vi "magTerm_TREEstate.vi"() -> ()   [LabVIEW 2014]
uses:
  <vilib>/Utility/file.llb/Read From Spreadsheet File (string).vi
  common/crest/LabVIEW/LV14/libcommon-crest.lvlib
panel:
  out "Waveform Chart":dbl[][](graph)
  out "current_buffer_array":dbl[][](array[numeric])
  out "array (last n elements first)":dbl[](array[numeric])
  in  "Tab Control":enum32{"Page 1", "Page 2"}(tab)
  out "handle":u32
  in  "Simulated/real":string(combo)="BTF_SIM"
  in  "Set_prog_state":bool
  in  "file path (dialog if empty)":path
  out "file_data":string[][](array[string])
  in  "stop":bool
  in  "!CHAOS WAN url":string="192.168.150.91:8081"
  out "Set_prog_Current":string[](array[string])
  out "RUN":bool
  out "Element List":string[](array[string])
  in  "buffer_size":i32=100
  out "function return":i32
  out "error":u32
  out "set_current_new":dbl
  out "set_current_new_control":string
  out "Array Element.Value":variant
  out "Timeout_Array":i64[](array[numeric])
  in  "Single MAG SETUP":T1
  out "MAG array display":T2(array[cluster])
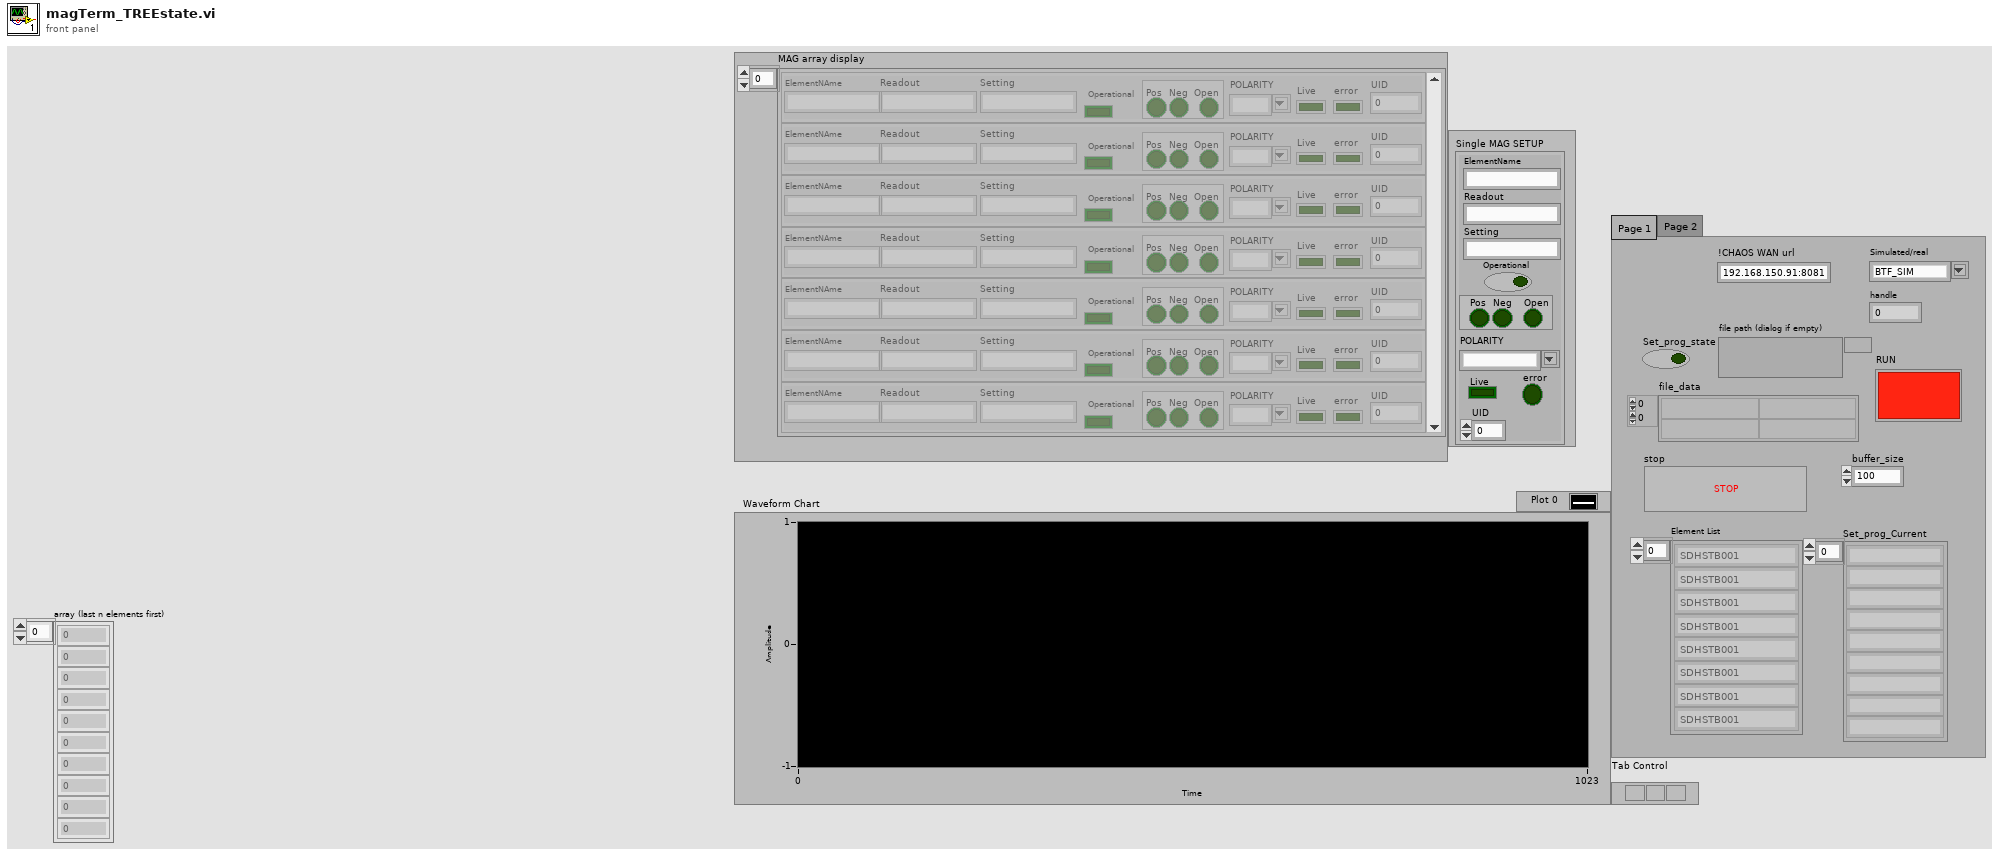
[diagram p1: front panel]
types:
  T1 = cluster{"ElementName":string, "Readout":string, "Setting":string, "Operational":bool, "Pos":bool, "Neg ":bool, "Open":bool, "Live":bool, "error":bool, "UID":u32, "POLARITY":string}
  T2 = cluster{"ElementNAme":string, "Readout":string, "Setting":string, "Operational":bool, "Pos":bool, "Neg ":bool, "Open":bool, "Live":bool, "error":bool, "UID":u32, "POLARITY":string}[]
  T3 = cluster{"ElementName":string, "Readout":string, "Setting":string, "Operational":bool, "Pos":bool, "Neg ":bool, "Open":bool, "Live":bool, "error":bool, "UID":u32, "POLARITY":string}[]
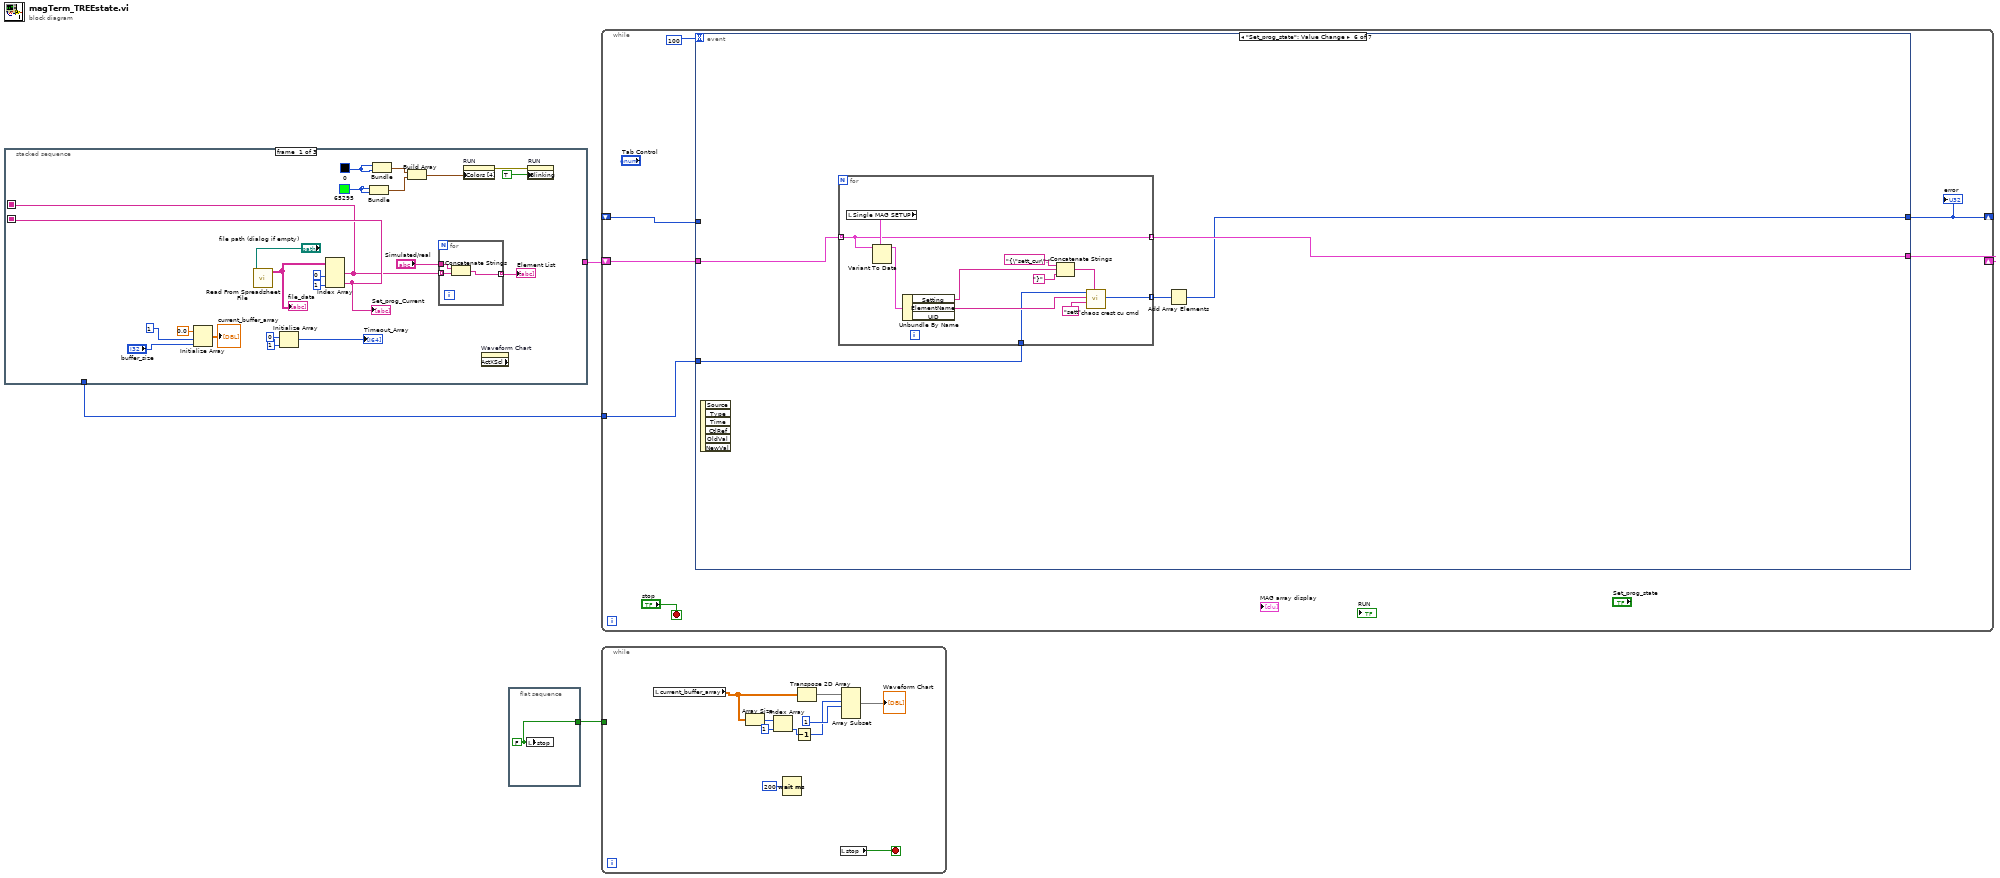
[diagram p0: block diagram]
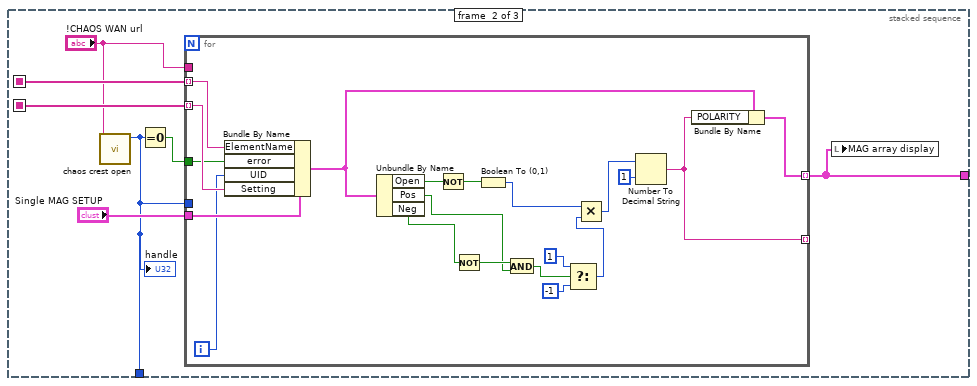
[diagram p2: hidden frame]
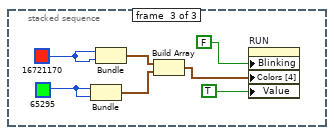
[diagram p3: hidden frame]
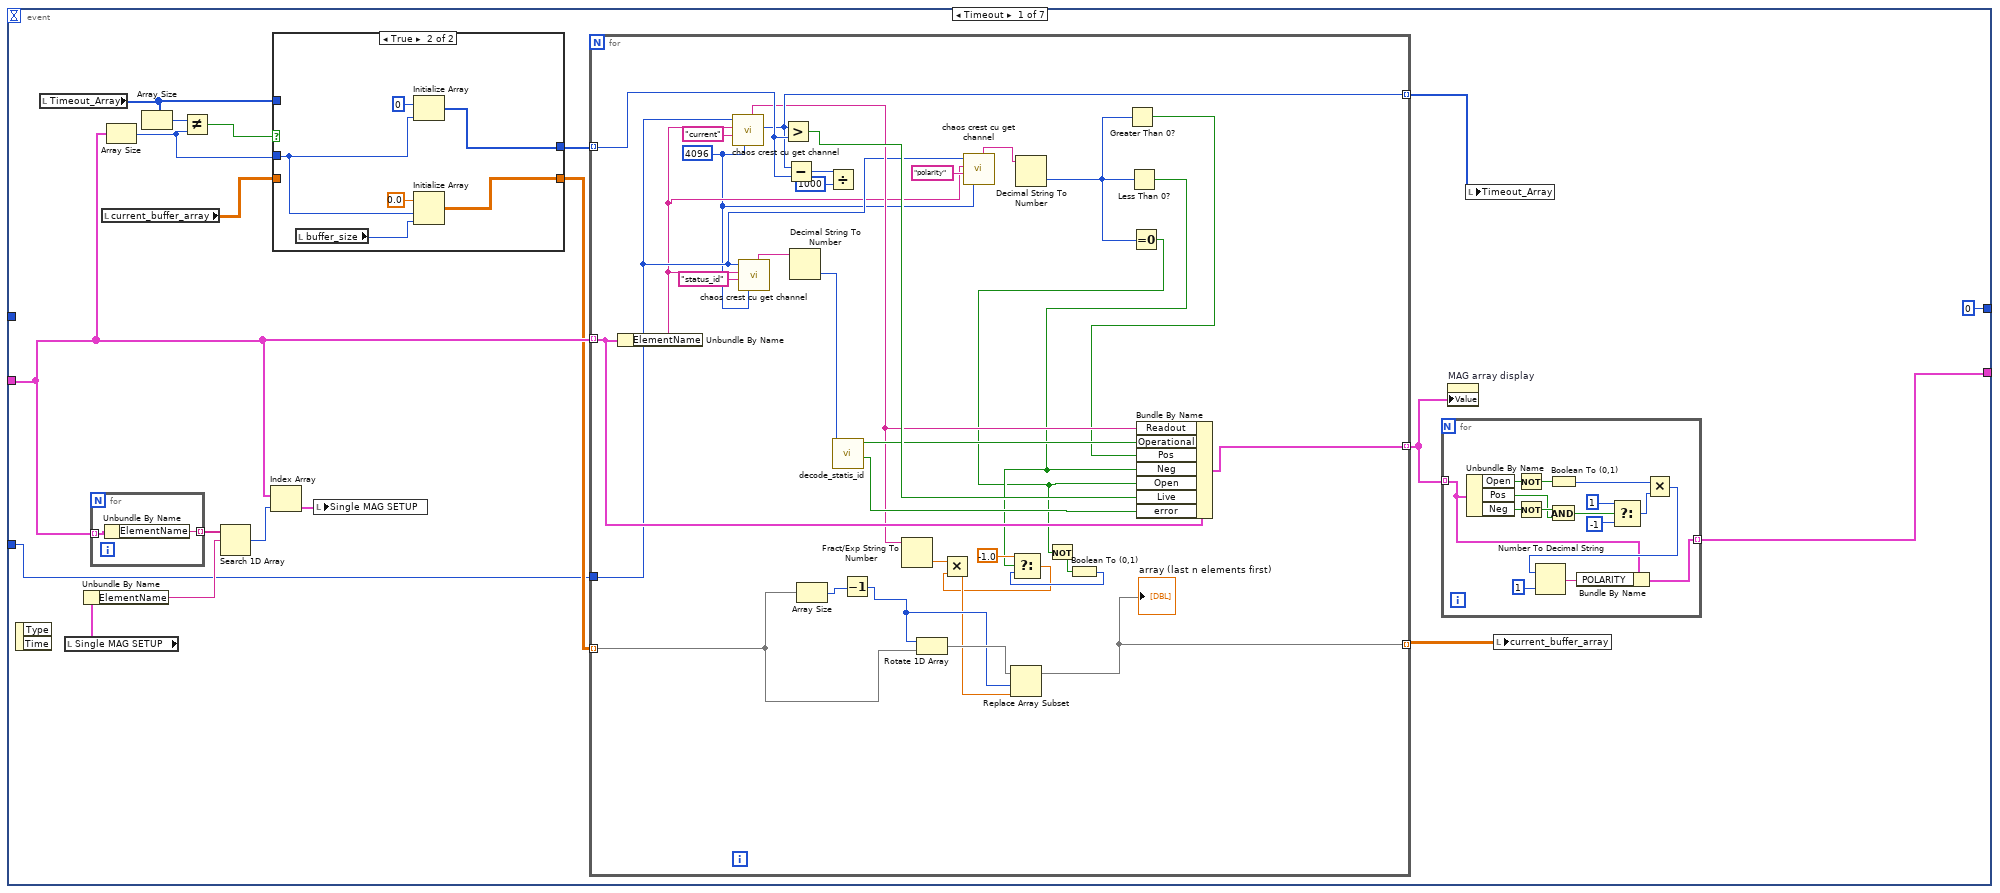
[diagram p4: hidden frame]
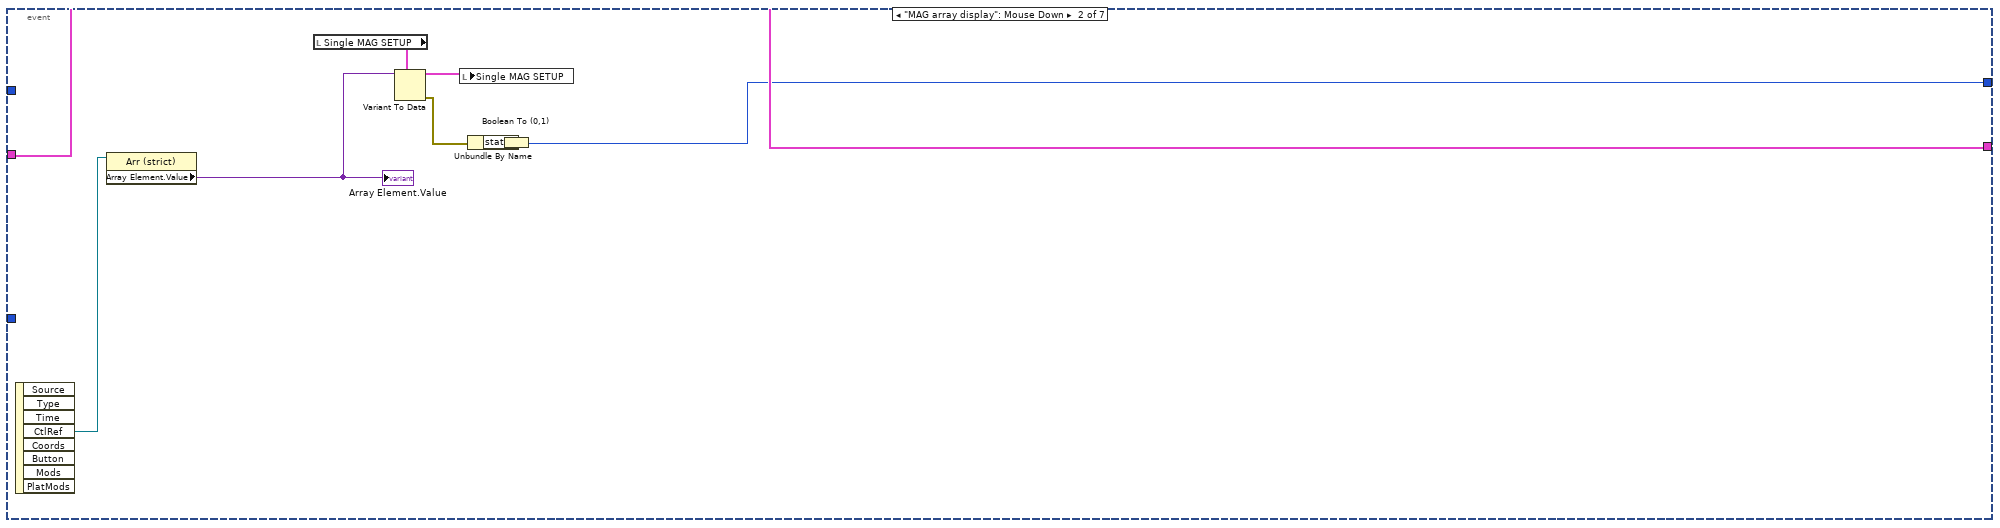
[diagram p6: hidden frame]
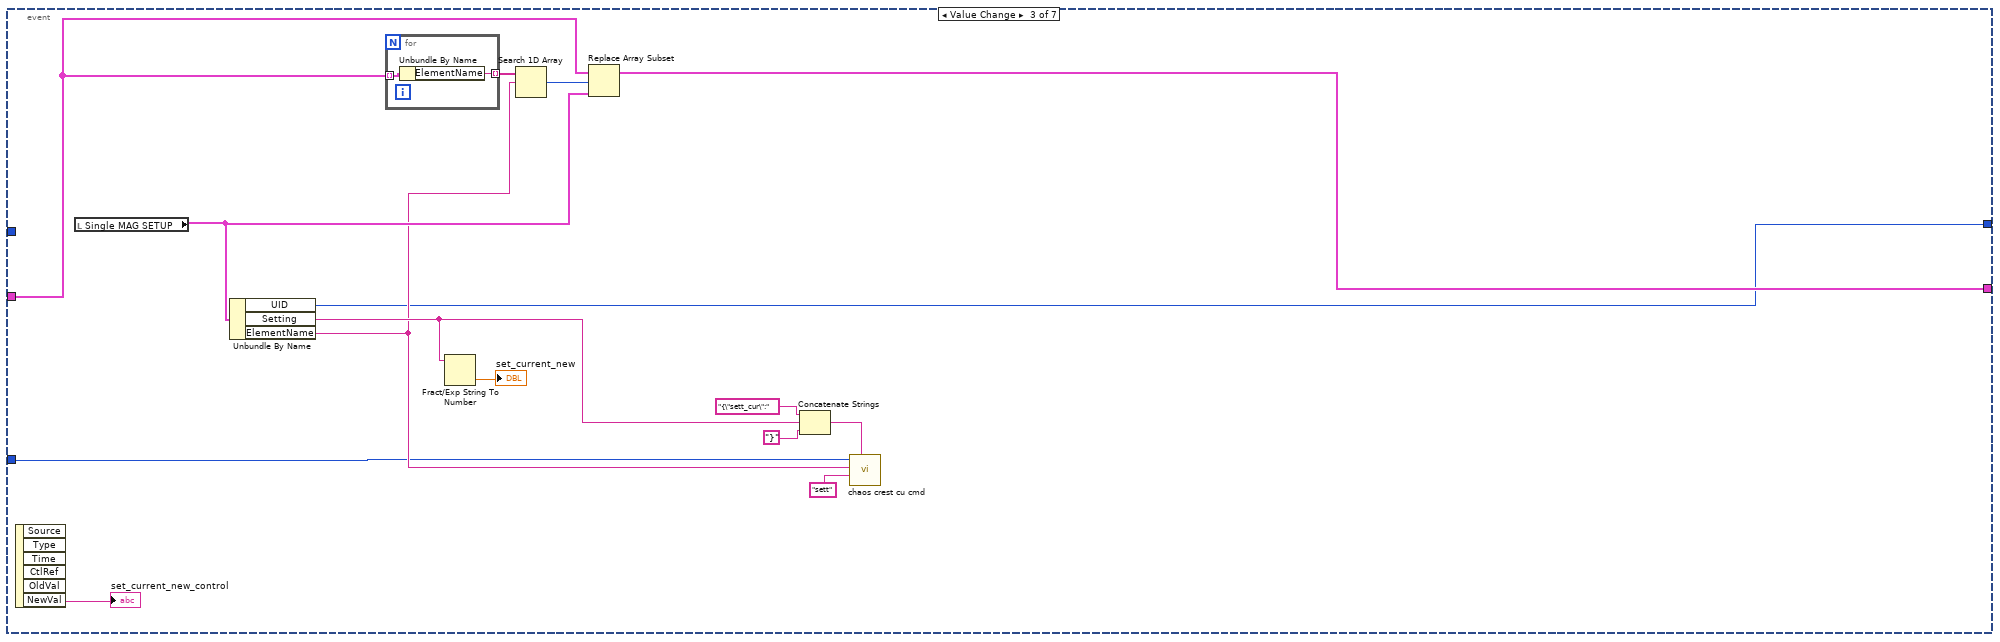
[diagram p7: hidden frame]
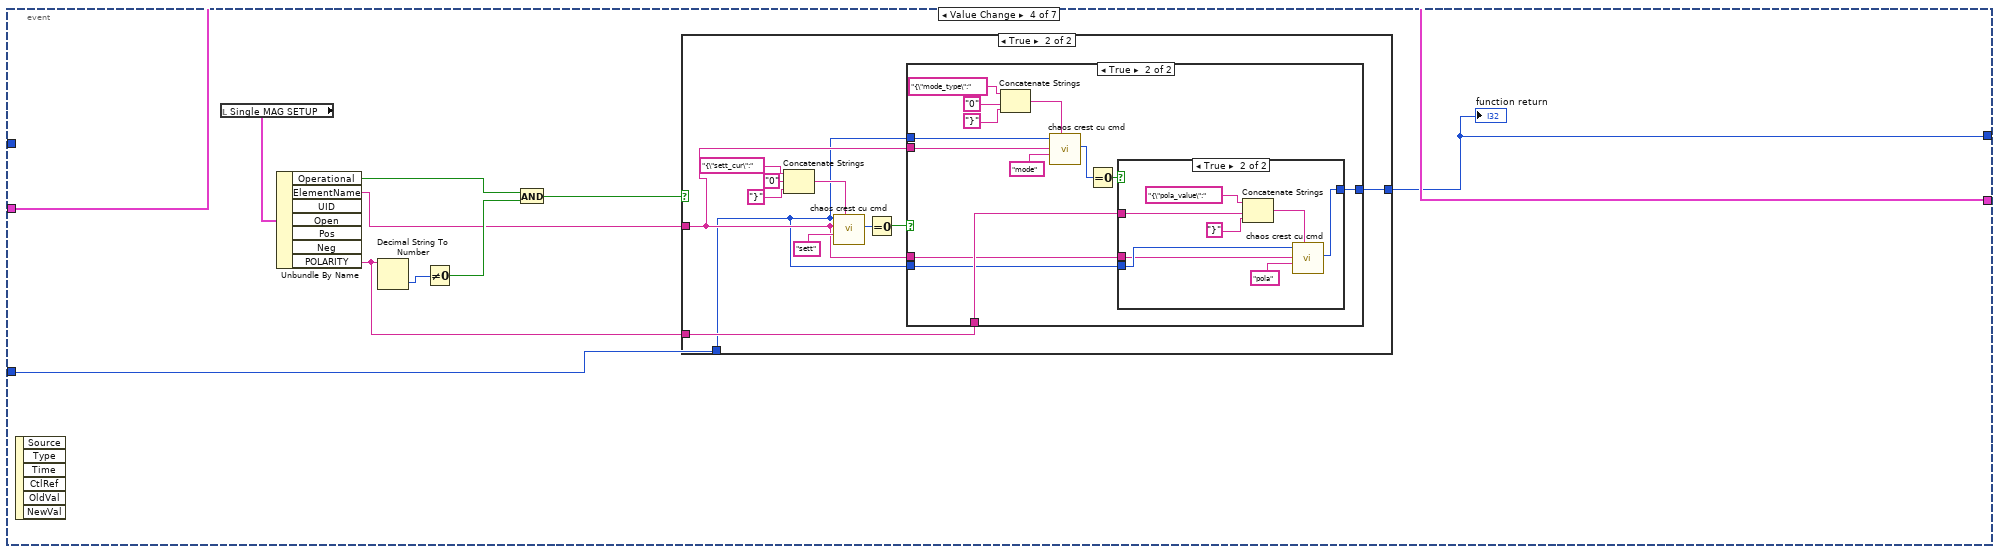
[diagram p8: hidden frame]
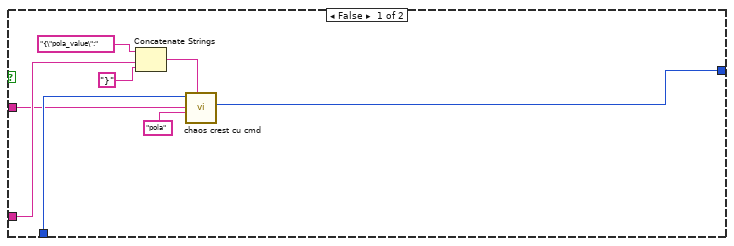
[diagram p9: hidden frame]
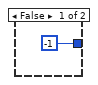
[diagram p10: hidden frame]
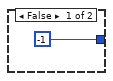
[diagram p11: hidden frame]
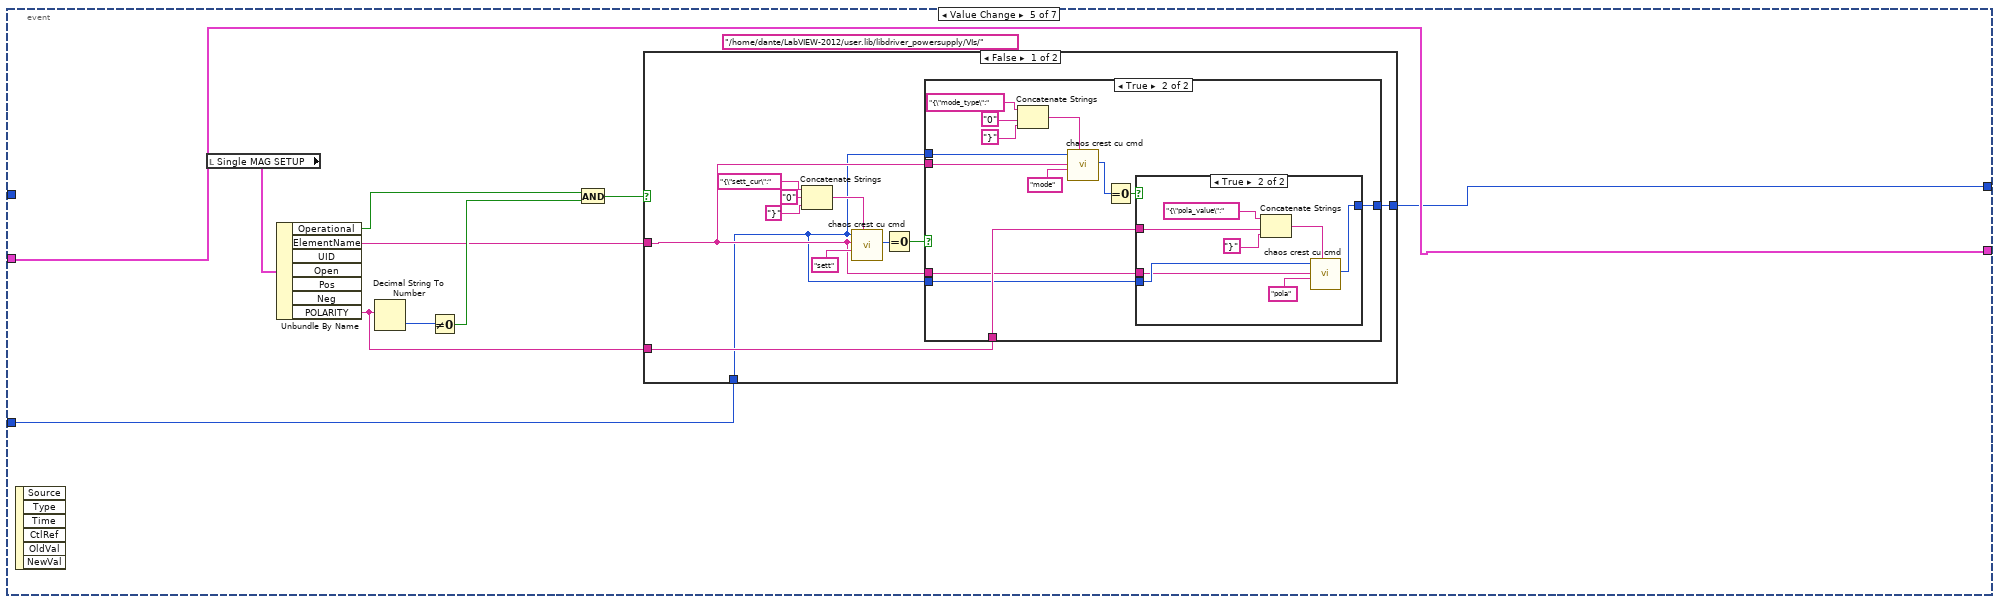
[diagram p12: hidden frame]
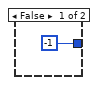
[diagram p13: hidden frame]
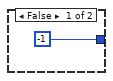
[diagram p14: hidden frame]
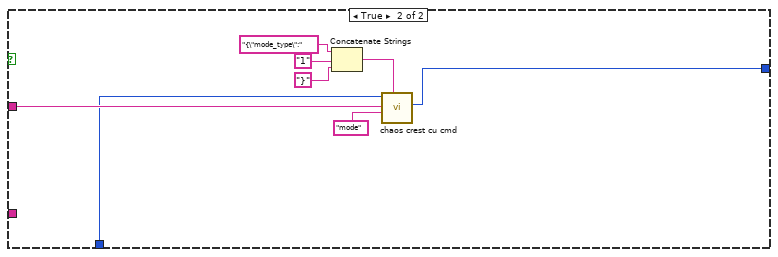
[diagram p15: hidden frame]
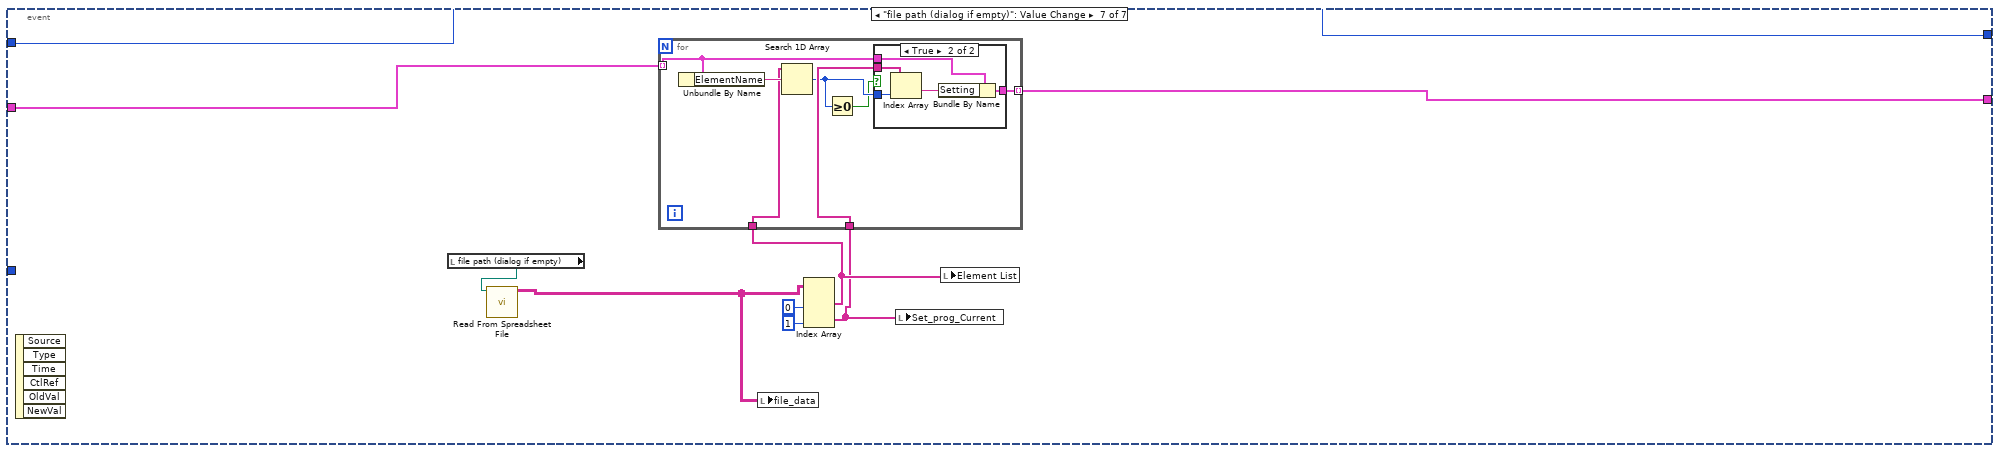
[diagram p16: hidden frame]
diagram:
  n1 = stacked-sequence {
    seq-local: [w6 _ _] -> [_ w35 _]
    seq-local: [w21 _ _] -> [_ w34 _]
    tunnel: [_ w33 _] -> w3
    tunnel: [_ w29 _] -> w1
    frame #0 {
      w17 = u32 0
      w16 = u32 65295
      n2 = Initialize Array(0.0 ("element"), 1 ("dimension size"), "buffer_size") -> (→"current_buffer_array":dbl[][])
      n3 = call-poly <vilib>:"Read From Spreadsheet File.vi"("file path (dialog if empty)"="file path (dialog if empty)") -> ("all rows"=w24:string[][])  [unwired: 6 in, 4 out]
      "file_data" <- w24
      n4 = Initialize Array(i64 0 ("element"), 1 ("dimension size")) -> (→"Timeout_Array":i64[])
      n5 = Index Array(array=w24, index (col) #1=0 ("disabled index (col)"), index (col) #2=1 ("index (col)")) -> (element #1=w6:string[], element #2=w21:string[])  [unwired: 2 in]
      "Set_prog_Current" <- w21
      n6 = Bundle(w16, w16) -> (w19:cluster{u32, u32})  [unwired: 1 in]
      n7 = Bundle(w17, w17) -> (w20:cluster{u32, u32})  [unwired: 1 in]
      n8 = Build Array(w20, w19) -> (w18:cluster{u32, u32}[])
      n9 = for {
        tunnel: w6 -> [w28] mode=indexing
        tunnel: "Simulated/real" -> [w27]
        tunnel: [w26] -> w4 mode=indexing
        n10 = Concatenate Strings(w27, w28) -> (w26:string)
      }
      "Element List" <- w4
      n11 = property on="RUN" class="Bool (strict)"("Colors [4]"=w18) -> (error out=w12:errorcluster)  [unwired: 2 in, 1 out]
      n12 = property on="Waveform Chart" class="WFChart (strict)" props=["ActXScl"]() -> ()  [unwired: 2 in, 3 out]
      n13 = property on="RUN" class="Bool (strict)"(error in=w12, "Blinking"=TRUE) -> ()  [unwired: 1 in, 2 out]
    }
    frame #1 {
      n14 = call "chaos crest open.vi"("chaoswanurl"="!CHAOS WAN url") -> ("function return"=w29:u32)  [unwired: 10 in]
      "handle" <- w29
      n15 = Equal To 0?(x=w29) -> (x = 0?=w30:bool)
      n16 = for {
        tunnel: w35 -> [w55] mode=indexing
        tunnel: "!CHAOS WAN url" -> [_]
        tunnel: [w39] -> w33 mode=indexing
        tunnel: w34 -> [w54] mode=indexing
        tunnel: "Single MAG SETUP" -> [w53]
        tunnel: [w38] -> _ mode=indexing
        tunnel: w30 -> [w36]
        tunnel: w29 -> [_]
        i -> [w37]
        n17 = Bundle By Name(cluster=w53, "ElementName"=w55, "error"=w36, "UID"=w37, "Setting"=w54) -> (w42:T1)
        n18 = Unbundle By Name(w42) -> ("Open"=w48:bool, "Pos"=w47:bool, "Neg"=w46:bool)
        n19 = Not(x=w48) -> (.not. x?=w45:bool)
        n20 = Not(x=w46) -> (.not. x?=w52:bool)
        n21 = Boolean To (0,1)(Boolean=w45) -> (0, 1=w44:i16)
        n22 = And(x=w52, y=w47) -> (x .and. y?=w51:bool)
        n23 = Select(t=1 ("pol"), s=w51, f=-1 ("pol")) -> (s? t:f=w43:i32)
        n24 = Multiply(x=w44, y=w43) -> (x*y=w41:i32)
        n25 = Number To Decimal String(number=w41, width (-)=i16 1) -> (decimal integer string=w38:string)
        n26 = Bundle By Name(cluster=w42, "POLARITY"=w38) -> (w39:T1)
      }
      n27 = local write "MAG array display"(w33) -> ()
    }
    frame #2 {
      w56 = u32 16721170
      w57 = u32 65295
      n28 = Bundle(w57, w57) -> (w61:cluster{u32, u32})  [unwired: 1 in]
      n29 = Bundle(w56, w56) -> (w62:cluster{u32, u32})  [unwired: 1 in]
      n30 = Build Array(w62, w61) -> (w60:cluster{u32, u32}[])
      n31 = property on="RUN" class="Bool (strict)"("Blinking"=FALSE, "Colors [4]"=w60, "Value"=TRUE) -> ()  [unwired: 2 in, 2 out]
    }
  }
  n32 = flat-sequence {
    tunnel: [w63] -> w2
    frame #0 {
      w63 = FALSE ("stop")
      n33 = local write "stop"(w63) -> ()
    }
  }
  n34 = while {
    shift-right: [w67] -> _
    shift-left: w3 -> [w68]
    shift-right: [w66] -> _
    shift-left: _ -> [w65]
    tunnel: w1 -> [w64]
    stop <- "stop" stop-if-true
    n35 = event shown="[5] \"Set_prog_state\": Value Change" {
      selector: _ -> [_ _ _ _ _ _ _]
      dyn-events: _ -> [_ _ _ _ _ _ _]
      timeout: 100 -> [_ _ _ _ _ _ _]
      tunnel: w68 -> [w80 w153 w168 w181 w233 w279 w299]
      tunnel: [w76 w153 w167 w181 w233 w282 w295] -> w67
      tunnel: [u32 0 ("UID") w149 w157 w180 w232 w280 w294] -> w66
      tunnel: w65 -> [_ _ _ _ _ _ w294]
      tunnel: w64 -> [w72 _ w158 w175 w227 w278 _]
      event Timeout {
        n36 = event-data() -> ()  [unwired: 1 in, 2 out]
        n37 = local read "Timeout_Array"() -> (w88:i64[])
        n38 = local read "Single MAG SETUP"() -> (w83:T1)
        n39 = Unbundle By Name(w83) -> ("ElementName"=w81:string)
        n40 = for {
          tunnel: w80 -> [w106] mode=indexing
          tunnel: [w105] -> w82 mode=indexing
          n41 = Unbundle By Name(w106) -> ("ElementName"=w105:string)
        }
        n42 = local read "current_buffer_array"() -> (w73:dbl[][])
        n43 = Array Size(array=w80) -> (size(s)=w85:i32)
        n44 = Array Size(array=w88) -> (size(s)=w87:i32)
        n45 = Not Equal?(x=w87, y=w85) -> (x != y?=w86:bool)
        n46 = Search 1D Array(1D array=w82, element=w81) -> (index of element=w79:i32)  [unwired: 1 in]
        n47 = Index Array(array=w80, index=w79) -> (element=w78:T1)
        n48 = case shown="True" w86 {
          tunnel: w88 -> [w108 _]
          tunnel: w85 -> [_ w110]
          tunnel: [w108 w113] -> w84
          tunnel: [w107 w111] -> w75
          tunnel: w73 -> [w107 _]
          frame False {
          }
          frame True {
            n49 = local read "buffer_size"() -> (w109:i32)
            n50 = Initialize Array(i64 0 ("element"), w110) -> (w113:i64[])
            n51 = Initialize Array(0.0 ("element"), w110, w109) -> (w111:dbl[][])
          }
        }
        n52 = local write "Single MAG SETUP"(w78) -> ()
        n53 = for {
          tunnel: w80 -> [w148] mode=indexing
          tunnel: [w147] -> w77 mode=indexing
          tunnel: [w132] -> w89 mode=indexing
          tunnel: w84 -> [w133] mode=indexing
          tunnel: w75 -> [w143] mode=indexing
          tunnel: [w142] -> w74 mode=indexing
          tunnel: w72 -> [w120]
          w118 = 4096 ("maxsize")
          n54 = Unbundle By Name(w148) -> ("ElementName"=w119:string)
          n55 = call "chaos crest cu get channel.vi"("maxsize"=w118, "channame"="current", "cuname"=w119, "h"=w120) -> ("timestamp"=w132:u64, "output out"=w125:string)  [unwired: 5 in, 1 out]
          n56 = call "chaos crest cu get channel.vi"("maxsize"=w118, "channame"="status_id", "cuname"=w119, "h"=w120) -> ("output out"=w130:string)  [unwired: 5 in, 2 out]
          n57 = Greater?(x=w132, y=w133) -> (0:w131:bool)
          n58 = Subtract(x=w132, y=w133) -> (x-y=w135:u64)
          n59 = Decimal String To Number(string=w130) -> (number=w128:i32)  [unwired: 2 in, 1 out]
          n60 = Array Size(array=w143) -> (size(s)=w146:i32)
          n61 = Divide(x=w135, y=u32 1000) -> ()  [unwired: 1 out]
          n62 = call "decode_statis_id.vi"("satatus_id"=w128) -> ("Error"=w126:bool, "Operational"=w127:bool)  [unwired: 7 in, 2 out]
          n63 = Decrement(x=w146) -> (x-1=w144:i32)
          n64 = Fract/Exp String To Number(string=w125) -> (number=w124:dbl)  [unwired: 3 in, 1 out]
          n65 = Rotate 1D Array(1:w143, 2:w144) -> (0:w145:dbl[])
          n66 = call "chaos crest cu get channel.vi"("maxsize"=w118, "channame"="polarity", "cuname"=w119, "h"=w120) -> ("output out"=w122:string)  [unwired: 5 in, 2 out]
          n67 = Decimal String To Number(string=w122) -> (number=w123:i32)  [unwired: 2 in, 1 out]
          n68 = Greater Than 0?(x=w123) -> (x > 0?=w117:bool)
          n69 = Less Than 0?(x=w123) -> (x < 0?=w116:bool)
          n70 = Equal To 0?(x=w123) -> (x = 0?=w115:bool)
          n71 = Not(x=w115) -> (.not. x?=w139:bool)
          n72 = Boolean To (0,1)(Boolean=w139) -> (0, 1=w138:i16)
          n73 = Select(t=-1.0, s=w116, f=w138) -> (s? t:f=w137:dbl)
          n74 = Multiply(x=w124, y=w137) -> (x*y=w141:dbl)
          n75 = Replace Array Subset(array=w145, new element=w141, index=w144) -> (w142:dbl[])
          "array (last n elements first)" <- w142
          n76 = Bundle By Name(cluster=w148, "Readout"=w125, "Operational"=w127, "Pos"=w117, "Neg"=w116, "Open"=w115, "Live"=w131, "error"=w126) -> (w147:T1)
        }
        n77 = for {
          tunnel: [w92] -> w76 mode=indexing
          tunnel: w77 -> [w90] mode=indexing
          n78 = Unbundle By Name(w90) -> ("Open"=w100:bool, "Pos"=w99:bool, "Neg"=w98:bool)
          n79 = Not(x=w100) -> (.not. x?=w97:bool)
          n80 = Not(x=w98) -> (.not. x?=w104:bool)
          n81 = Boolean To (0,1)(Boolean=w97) -> (0, 1=w96:i16)
          n82 = And(x=w104, y=w99) -> (x .and. y?=w103:bool)
          n83 = Select(t=1 ("pol"), s=w103, f=-1 ("pol")) -> (s? t:f=w95:i32)
          n84 = Multiply(x=w96, y=w95) -> (x*y=w94:i32)
          n85 = Number To Decimal String(number=w94, width (-)=i16 1) -> (decimal integer string=w91:string)
          n86 = Bundle By Name(cluster=w90, "POLARITY"=w91) -> (w92:T1)
        }
        n87 = property on="MAG array display" class="Arr (strict)"("Value"=w77) -> ()  [unwired: 2 in, 2 out]
        n88 = local write "Timeout_Array"(w89) -> ()
        n89 = local write "current_buffer_array"(w74) -> ()
      }
      event "MAG array display": Mouse Down {
        n90 = event-data() -> ("CtlRef"=w156:refnum<vi>)  [unwired: 1 in, 7 out]
        n91 = property class="Arr (strict)"(reference=w156) -> ("Array Element.Value"=w155:variant)  [unwired: 1 in, 2 out]
        "Array Element.Value" <- w155
        n92 = local read "Single MAG SETUP"() -> (w154:T1)
        n93 = Variant To Data(type=w154, Variant=w155) -> (data=w152:T1, error out=w151:errorcluster)  [unwired: 1 in]
        n94 = local write "Single MAG SETUP"(w152) -> ()
        n95 = Unbundle By Name(w151) -> ("status"=w150:bool)
        n96 = Boolean To (0,1)(Boolean=w150) -> (0, 1=w149:i16)
      }
      event "Single MAG SETUP.Setting": Value Change {
        n97 = event-data() -> ("NewVal"=→"set_current_new_control":string)  [unwired: 1 in, 5 out]
        n98 = local read "Single MAG SETUP"() -> (w166:T1)
        n99 = Unbundle By Name(w166) -> ("UID"=w157:u32, "Setting"=w160:string, "ElementName"=w159:string)
        n100 = for {
          tunnel: w168 -> [w173] mode=indexing
          tunnel: [w172] -> w170 mode=indexing
          n101 = Unbundle By Name(w173) -> ("ElementName"=w172:string)
        }
        n102 = Fract/Exp String To Number(string=w160) -> (number=→"set_current_new":dbl)  [unwired: 3 in, 1 out]
        n103 = Search 1D Array(1D array=w170, element=w159) -> (index of element=w169:i32)  [unwired: 1 in]
        n104 = Replace Array Subset(array=w168, new element=w166, index=w169) -> (w167:T3)
        n105 = Concatenate Strings("{\"sett_cur\":", w160, "}" ("string")) -> (w163:string)
        n106 = call "chaos crest cu cmd.vi"("args"=w163, "cmd"="sett", "cuname"=w159, "h"=w158) -> ()  [unwired: 6 in, 2 out]
      }
      event "Single MAG SETUP.POLARITY": Value Change {
        n107 = event-data() -> ()  [unwired: 1 in, 6 out]
        n108 = local read "Single MAG SETUP"() -> (w183:T1)
        n109 = Unbundle By Name(w183) -> ("Operational"=w182:bool, "ElementName"=w176:string, "POLARITY"=w174:string)  [unwired: 4 out]
        n110 = Decimal String To Number(string=w174) -> (number=w179:i32)  [unwired: 2 in, 1 out]
        n111 = Not Equal To 0?(x=w179) -> (x != 0?=w178:bool)
        n112 = And(x=w182, y=w178) -> (x .and. y?=w177:bool)
        n113 = case shown="True" w177 {
          tunnel: [w184 w202] -> w180
          tunnel: w176 -> [w185 w193]
          tunnel: w175 -> [w186 w192]
          tunnel: w174 -> [w187 w194]
          frame False {
            n114 = Concatenate Strings("{\"pola_value\":", w187, "}" ("string")) -> (w190:string)
            n115 = call "chaos crest cu cmd.vi"("args"=w190, "cmd"="pola", "cuname"=w185, "h"=w186) -> ("function return"=w184:i32)  [unwired: 6 in, 1 out]
          }
          frame True {
            n116 = Concatenate Strings("{\"sett_cur\":", "0" ("string"), "}" ("string")) -> (w200:string)
            n117 = call "chaos crest cu cmd.vi"("args"=w200, "cmd"="sett", "cuname"=w193, "h"=w192) -> ("function return"=w196:i32)  [unwired: 6 in, 1 out]
            n118 = Equal To 0?(x=w196) -> (x = 0?=w195:bool)
            n119 = case shown="True" w195 {
              tunnel: [-1 ("function return") w215] -> w202
              tunnel: w194 -> [_ w214]
              tunnel: w192 -> [_ w213]
              tunnel: w193 -> [_ w212]
              tunnel: w193 -> [_ w205]
              tunnel: w192 -> [_ w204]
              frame False {
              }
              frame True {
                n120 = Concatenate Strings("{\"mode_type\":", "0" ("string"), "}" ("string")) -> (w209:string)
                n121 = call "chaos crest cu cmd.vi"("args"=w209, "cmd"="mode", "cuname"=w205, "h"=w204) -> ("function return"=w206:i32)  [unwired: 6 in, 1 out]
                n122 = Equal To 0?(x=w206) -> (x = 0?=w216:bool)
                n123 = case shown="True" w216 {
                  tunnel: [-1 ("function return") w218] -> w215
                  tunnel: w214 -> [_ w222]
                  tunnel: w213 -> [_ w220]
                  tunnel: w212 -> [_ w219]
                  frame False {
                  }
                  frame True {
                    n124 = Concatenate Strings("{\"pola_value\":", w222, "}" ("string")) -> (w224:string)
                    n125 = call "chaos crest cu cmd.vi"("args"=w224, "cmd"="pola", "cuname"=w219, "h"=w220) -> ("function return"=w218:i32)  [unwired: 6 in, 1 out]
                  }
                }
              }
            }
          }
        }
        "function return" <- w180
      }
      event "Single MAG SETUP.Operational": Value Change {
        (unwired) "/home/dante/LabVIEW-2012/user.lib/libdriver_powersupply/VIs/"
        n126 = event-data() -> ()  [unwired: 1 in, 6 out]
        n127 = local read "Single MAG SETUP"() -> (w235:T1)
        n128 = Unbundle By Name(w235) -> ("Operational"=w234:bool, "ElementName"=w228:string, "POLARITY"=w226:string)  [unwired: 4 out]
        n129 = Decimal String To Number(string=w226) -> (number=w229:i32)  [unwired: 2 in, 1 out]
        n130 = Not Equal To 0?(x=w229) -> (x != 0?=w231:bool)
        n131 = And(x=w234, y=w231) -> (x .and. y?=w230:bool)
        n132 = case shown="False" w230 {
          tunnel: [w236 w272] -> w232
          tunnel: w228 -> [w239 w271]
          tunnel: w227 -> [w237 w270]
          tunnel: w226 -> [w238 _]
          frame False {
            n133 = Concatenate Strings("{\"sett_cur\":", "0" ("string"), "}" ("string")) -> (w245:string)
            n134 = call "chaos crest cu cmd.vi"("args"=w245, "cmd"="sett", "cuname"=w239, "h"=w237) -> ("function return"=w241:i32)  [unwired: 6 in, 1 out]
            n135 = Equal To 0?(x=w241) -> (x = 0?=w240:bool)
            n136 = case shown="True" w240 {
              tunnel: [-1 ("function return") w259] -> w236
              tunnel: w238 -> [_ w258]
              tunnel: w237 -> [_ w257]
              tunnel: w239 -> [_ w256]
              tunnel: w239 -> [_ w249]
              tunnel: w237 -> [_ w248]
              frame False {
              }
              frame True {
                n137 = Concatenate Strings("{\"mode_type\":", "0" ("string"), "}" ("string")) -> (w253:string)
                n138 = call "chaos crest cu cmd.vi"("args"=w253, "cmd"="mode", "cuname"=w249, "h"=w248) -> ("function return"=w250:i32)  [unwired: 6 in, 1 out]
                n139 = Equal To 0?(x=w250) -> (x = 0?=w260:bool)
                n140 = case shown="True" w260 {
                  tunnel: [-1 ("function return") w262] -> w259
                  tunnel: w258 -> [_ w266]
                  tunnel: w257 -> [_ w264]
                  tunnel: w256 -> [_ w263]
                  frame False {
                  }
                  frame True {
                    n141 = Concatenate Strings("{\"pola_value\":", w266, "}" ("string")) -> (w268:string)
                    n142 = call "chaos crest cu cmd.vi"("args"=w268, "cmd"="pola", "cuname"=w263, "h"=w264) -> ("function return"=w262:i32)  [unwired: 6 in, 1 out]
                  }
                }
              }
            }
          }
          frame True {
            n143 = Concatenate Strings("{\"mode_type\":", "1" ("string"), "}" ("string")) -> (w275:string)
            n144 = call "chaos crest cu cmd.vi"("args"=w275, "cmd"="mode", "cuname"=w271, "h"=w270) -> ("function return"=w272:i32)  [unwired: 6 in, 1 out]
          }
        }
      }
      event "Set_prog_state": Value Change {
        n145 = event-data() -> ()  [unwired: 1 in, 6 out]
        n146 = for {
          tunnel: w279 -> [w291] mode=indexing
          tunnel: [w291] -> w282 mode=indexing
          tunnel: [w284] -> w281 mode=indexing
          tunnel: w278 -> [w285]
          n147 = local read "Single MAG SETUP"() -> (w292:T1)
          n148 = Variant To Data(type=w292, Variant=w291) -> (data=w293:T1)  [unwired: 1 in, 1 out]
          n149 = Unbundle By Name(w293) -> ("Setting"=w287:string, "ElementName"=w286:string)  [unwired: 1 out]
          n150 = Concatenate Strings("{\"sett_cur\":", w287, "}" ("string")) -> (w289:string)
          n151 = call "chaos crest cu cmd.vi"("args"=w289, "cmd"="sett", "cuname"=w286, "h"=w285) -> ("function return"=w284:i32)  [unwired: 6 in, 1 out]
        }
        n152 = Add Array Elements(numeric array=w281) -> (sum=w280:i32)
      }
      event "file path (dialog if empty)": Value Change {
        n153 = event-data() -> ()  [unwired: 1 in, 6 out]
        n154 = local read "file path (dialog if empty)"() -> (w302:path)
        n155 = call-poly <vilib>:"Read From Spreadsheet File.vi"("file path (dialog if empty)"=w302) -> ("all rows"=w298:string[][])  [unwired: 6 in, 4 out]
        n156 = local write "file_data"(w298) -> ()
        n157 = Index Array(array=w298, index (col) #1=0 ("disabled index (col)"), index (col) #2=1 ("index (col)")) -> (element #1=w297:string[], element #2=w296:string[])  [unwired: 2 in]
        n158 = for {
          tunnel: w299 -> [w306] mode=indexing
          tunnel: w297 -> [w308]
          tunnel: w296 -> [w307]
          tunnel: [w305] -> w295 mode=indexing
          n159 = Unbundle By Name(w306) -> ("ElementName"=w309:string)
          n160 = Search 1D Array(1D array=w308, element=w309) -> (index of element=w304:i32)  [unwired: 1 in]
          n161 = Greater Or Equal To 0?(x=w304) -> (x >= 0?=w303:bool)
          n162 = case shown="True" w303 {
            tunnel: w307 -> [_ w315]
            tunnel: w304 -> [_ w314]
            tunnel: w306 -> [w310 w313]
            tunnel: [w310 w311] -> w305
            frame False {
            }
            frame True {
              n163 = Index Array(array=w315, index=w314) -> (element=w312:string)
              n164 = Bundle By Name(cluster=w313, "Setting"=w312) -> (w311:T1)
            }
          }
        }
        n165 = local write "Set_prog_Current"(w296) -> ()
        n166 = local write "Element List"(w297) -> ()
      }
    }
    "error" <- w66
  }
  n167 = while {
    tunnel: w2 -> [_]
    stop <- w325 stop-if-true
    n168 = local read "current_buffer_array"() -> (w320:dbl[][])
    n169 = Array Size(array=w320) -> (size(s)=w319:i32[])
    n170 = Index Array(array=w319, index=1) -> (element=w317:i32)
    n171 = Wait (ms)(milliseconds to wait=u32 200) -> ()  [unwired: 1 out]
    n172 = Decrement(x=w317) -> (x-1=w316:i32)
    n173 = Transpose 2D Array(2D array=w320) -> (transposed array=w323:dbl[][])
    n174 = local read "stop"() -> (w325:bool)
    n175 = Array Subset(array=w323, index (row)=w316, length (row)=1 ("length")) -> (→"Waveform Chart":dbl[][])  [unwired: 2 in]
  }
